vi "Tag.last_lua.vi"(5 "LuaVIEW reference":T1) -> (15 "error out":errorcluster)   [LabVIEW 2012]
doc: "Reads the last point written to the tag from its in-memory buffer. On initialisation, the datalogger rebuffers the last point which is therefore guaranteed to be available.\nParameters:\nobj:tag\nResults:\nnum:value, value of last written point.\nnum:time, timestamp of last written point.\nErrors:\nDead or invalid tag object.\nData logger not initialized."
uses:
  luaview/typedefs/t_LuaVIEW Reference.ctl
  typedefs/t_DataLog Tag Buffers Methods.ctl
  luaview/subvis/private/LuaVIEW Pull (object).vi
  luaview/subvis/private/LuaVIEW Push (number).vi
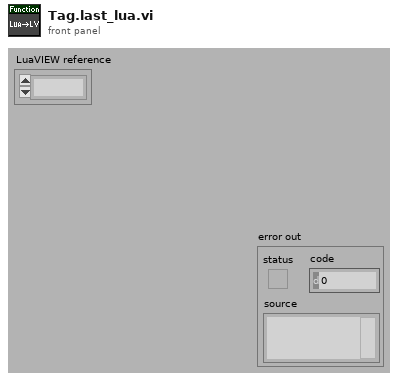
[diagram p1: front panel]
types:
  T1 = typedef "t_LuaVIEW Reference.ctl" = refnum<k1>
  T2 = typedef "t_DataLog Tag Buffers Methods.ctl" = enum16{"initialize", "inert", "write", "read", "read oldest", "read last", "cleanup"}
  T3 = typedef "t_DataLog Point.ctl" = cluster{"time":dbl, "value":dbl}
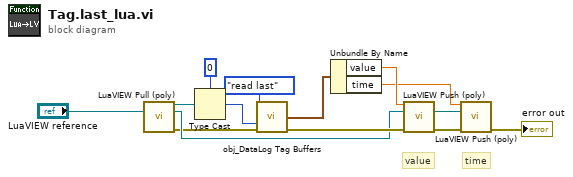
[diagram p0: block diagram]
diagram:
  # "time"
  # "value"
  n1 = call-poly "LuaVIEW Pull (poly).vi"("LuaVIEW reference in"="LuaVIEW reference") -> ("object refnum"=w8:refnum<vi>, "LuaVIEW reference out"=w11:T1, "error out"=w10:errorcluster)  [unwired: 11 in, 1 out]
  n2 = Type Cast(type=0 ("read index in"), x=w8) -> (*(type *) &x=w6:i32)
  n3 = call "obj_DataLog Tag Buffers.vi"("method"=t_DataLog_Tag_Buffers_Methods."read last", "tag index"=w6, "error in (no error)"=w10) -> ("point out"=w13:T3, "error out"=w12:errorcluster)  [unwired: 8 in, 3 out]
  n4 = Unbundle By Name(w13) -> ("value"=w3:dbl, "time"=w2:dbl)
  n5 = call-poly "LuaVIEW Push (poly).vi"("number"=w3, "LuaVIEW reference in"=w11, "error in (no error)"=w12) -> ("LuaVIEW reference out"=w4:T1, "error out"=w1:errorcluster)  [unwired: 11 in]
  n6 = call-poly "LuaVIEW Push (poly).vi"("number"=w2, "LuaVIEW reference in"=w4, "error in (no error)"=w1) -> ("error out"=→"error out":errorcluster)  [unwired: 11 in, 1 out]
